vi "test_RPLiDAR_Main3.vi"() -> ()   [LabVIEW 2019]
uses:
  Ctrl/rplidar_cmd.ctl
panel:
  out "XY Graph 4":cluster{"X":dbl, "Y":dbl}[](graph)=[{"X"=0.2824515072806151, "Y"=0.6855971091208806}, {"X"=0.2973493100074656, "Y"=0.6926199898487512}, {"X"=0.3182824081797592, "Y"=0.6879391751043789}, {"X"=0.32968595340345086, "Y"=0.6878188239852538}, {"X"=0.37688086730076775, "Y"=0.6851896174509806}, {"X"=0.423959702735745, "Y"=0.6772438042951879}, {"X"=0.10556803270784879, "Y"=0.0575799702170344}, {"X"=0.12764458907753945, "Y"=0.07189651507010685}, {"X"=0.162706267337329, "Y"=0.09217196194696962}, {"X"=0.5750904329426066, "Y"=0.3543603306493057}, {"X"=1.029570390073907, "Y"=0.5877032090120513}, {"X"=1.0369879212881827, "Y"=0.5729647577315851}, {"X"=1.0389160564866784, "Y"=0.5542198819730025}, {"X"=1.030226109276704, "Y"=0.530956837948797}, {"X"=1.0296780247760362, "Y"=0.5126775085697838}, {"X"=1.022823338060012, "Y"=0.49026062621811095}, {"X"=1.025782655226549, "Y"=0.47458930322582177}, {"X"=1.0232750025025923, "Y"=0.45592579632361235}, {"X"=1.026310539216213, "Y"=0.4396122462963535}, {"X"=1.0220381799563654, "Y"=0.4207321252429865}, {"X"=1.0194214725289468, "Y"=0.40316736456081603}, {"X"=1.0201040780016217, "Y"=0.386164773826486}, {"X"=0.9777644288999799, "Y"=0.3543680594775664}, {"X"=0.981222843840791, "Y"=0.33935938652848674}, {"X"=0.9788143096363876, "Y"=0.32306053573756427}]
  out "x != 0?":bool
  in  "Boolean":bool
  in  "Tab Control":enum32{"UI", "ref"}(tab)
  out "buffer":u32(graph)
  in  "Reset":bool
  in  "port":refnum<visa-resource-name>="COM6"
  in  "baud rate":u32=115200
  in  "stop":bool
  out "dt_check":u32=20
  out "rs232 data":string
  in  "dt":u32=20
  out "response check":bool=TRUE
  out "n_enq":i32=10469
  out "n q buf":i32
  out "element":string
  in  "Reset data":bool=TRUE
  out "real packet":bool
  in  "scan":bool
  in  "health":bool
  in  "stop":bool
  in  "spin":bool
  out "health check":bool
  in  "close":bool
  out "XY Graph 3":cluster{"X":dbl, "Y":dbl}[](graph)=[{"X"=0.2824515072806151, "Y"=0.6855971091208806}, {"X"=0.2973493100074656, "Y"=0.6926199898487512}, {"X"=0.3182824081797592, "Y"=0.6879391751043789}, {"X"=0.32968595340345086, "Y"=0.6878188239852538}, {"X"=0.37688086730076775, "Y"=0.6851896174509806}, {"X"=0.423959702735745, "Y"=0.6772438042951879}, {"X"=0.10556803270784879, "Y"=0.0575799702170344}, {"X"=0.12764458907753945, "Y"=0.07189651507010685}, {"X"=0.162706267337329, "Y"=0.09217196194696962}, {"X"=0.5750904329426066, "Y"=0.3543603306493057}, {"X"=1.029570390073907, "Y"=0.5877032090120513}, {"X"=1.0369879212881827, "Y"=0.5729647577315851}, {"X"=1.0389160564866784, "Y"=0.5542198819730025}, {"X"=1.030226109276704, "Y"=0.530956837948797}, {"X"=1.0296780247760362, "Y"=0.5126775085697838}, {"X"=1.022823338060012, "Y"=0.49026062621811095}, {"X"=1.025782655226549, "Y"=0.47458930322582177}, {"X"=1.0232750025025923, "Y"=0.45592579632361235}, {"X"=1.026310539216213, "Y"=0.4396122462963535}, {"X"=1.0220381799563654, "Y"=0.4207321252429865}, {"X"=1.0194214725289468, "Y"=0.40316736456081603}, {"X"=1.0201040780016217, "Y"=0.386164773826486}, {"X"=0.9777644288999799, "Y"=0.3543680594775664}, {"X"=0.981222843840791, "Y"=0.33935938652848674}, {"X"=0.9788143096363876, "Y"=0.32306053573756427}]
  out "update":bool
  out "read buffer":string
  out "unsigned byte array 2":u8[][](array[numeric]) format="%02x"
  # "RPLIDAR"
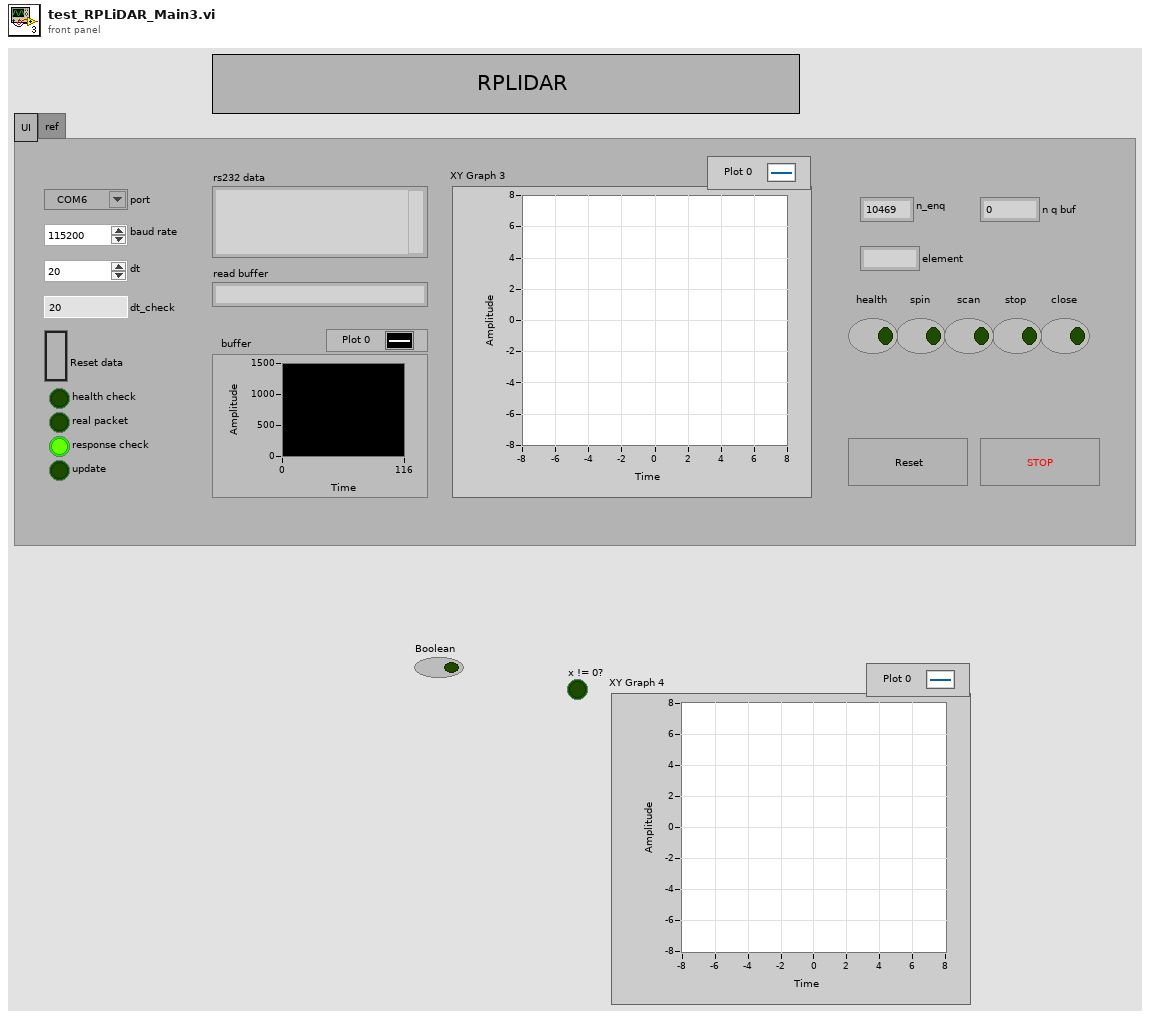
[diagram p1: front panel]
types:
  T1 = typedef "rplidar_cmd.ctl" = enum16{"init", "health", "spin", "scan", "read", "stop", "close"}
  T2 = cluster{"port":refnum<visa-resource-name>, "dt":u32, "update n":u8, "speed":u16, "rate ":u32}
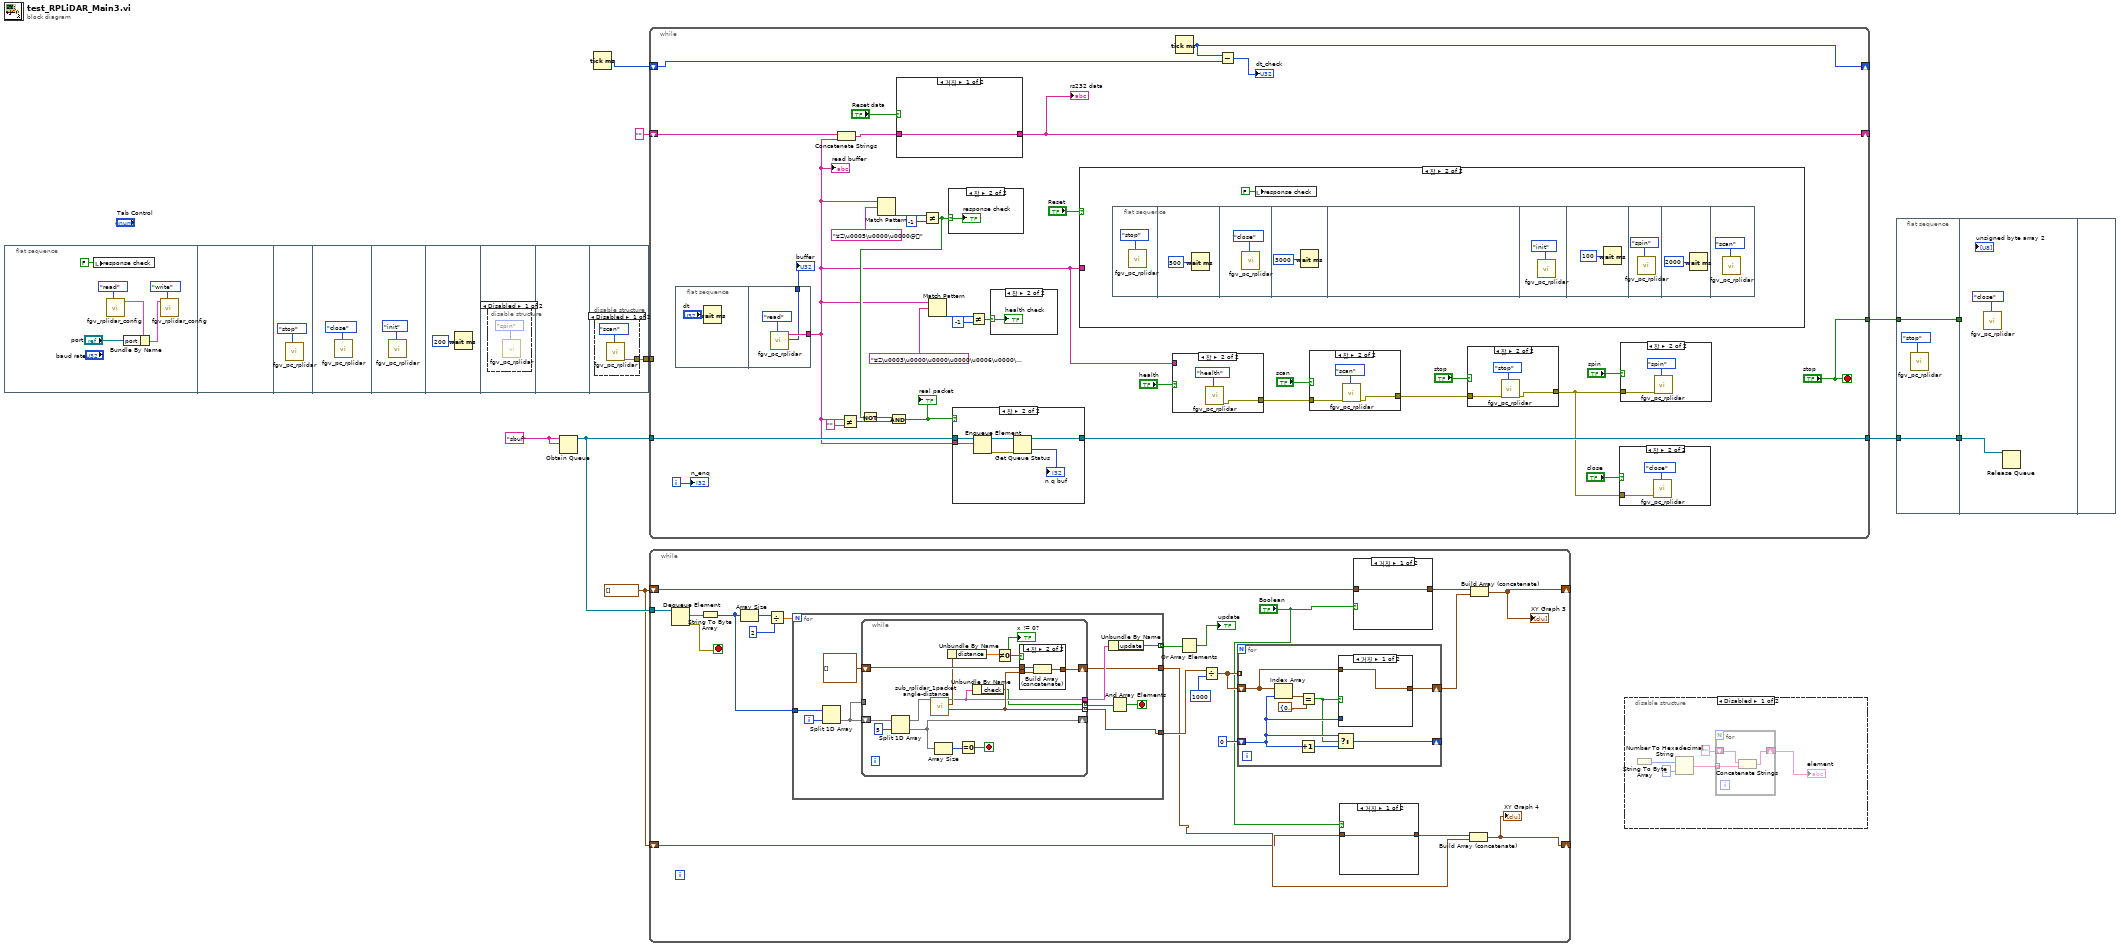
[diagram p0: block diagram]
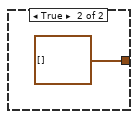
[diagram p3: hidden frame]
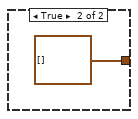
[diagram p4: hidden frame]
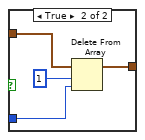
[diagram p5: hidden frame]
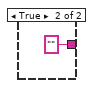
[diagram p15: hidden frame]
diagram:
  w1 = cluster{dbl, dbl}[] []
  w7 = "sbuf" ("name (unnamed)")
  n1 = flat-sequence {
    tunnel: [w22] -> w9
    frame #0 {
      n2 = local write "response check"(FALSE ("response check")) -> ()
      n3 = call "fgv_rplidar_config.vi"("cmd"=enum16{"read", "write"}."read") -> ("RPLidar cfg out"=w13:T2)  [unwired: 9 in, 1 out]
      n4 = Bundle By Name(cluster=w13, "port"="port") -> (w11:T2)
      n5 = call "fgv_rplidar_config.vi"("cmd"=enum16{"read", "write"}."write", "RPLidar cfg"=w11) -> ()  [unwired: 8 in, 2 out]
    }
    frame #1 {
    }
    frame #2 {
      n6 = call "fgv_pc_rplidar.vi"("cmd"=rplidar_cmd."stop") -> ()  [unwired: 8 in, 3 out]
    }
    frame #3 {
      n7 = call "fgv_pc_rplidar.vi"("cmd"=rplidar_cmd."close") -> ()  [unwired: 8 in, 3 out]
    }
    frame #4 {
      n8 = call "fgv_pc_rplidar.vi"("cmd"=rplidar_cmd."init") -> ()  [unwired: 8 in, 3 out]
    }
    frame #5 {
      n9 = Wait (ms)(milliseconds to wait=u32 200) -> ()  [unwired: 1 out]
    }
    frame #6 {
      n10 = disable-structure shown="Disabled" {
        frame Disabled {
          n11 = call "fgv_pc_rplidar.vi"("cmd"=rplidar_cmd."spin") -> ()  [unwired: 8 in, 3 out]
        }
        frame Enabled {
        }
      }
    }
    frame #7 {
    }
    frame #8 {
      n12 = disable-structure shown="Disabled" {
        disable-tunnel: [w23 _] -> w22
        frame Disabled {
          n13 = call "fgv_pc_rplidar.vi"("cmd"=rplidar_cmd."scan") -> ("error out"=w23:errorcluster)  [unwired: 8 in, 2 out]
        }
        frame Enabled {
        }
      }
    }
  }
  n14 = Obtain Queue(name (unnamed)=w7, element data type=w7) -> (queue out=w2:refnum<queue>)  [unwired: 3 in, 2 out]
  n15 = Tick Count (ms)() -> (millisecond timer value=w8:u32)
  n16 = while {
    tunnel: ["stop"] -> w10
    tunnel: w9 -> [_]
    shift-right: [w55] -> _
    shift-left: w8 -> [w54]
    shift-right: [w42] -> _
    shift-left: "" -> [w53]
    tunnel: w2 -> [w47]
    tunnel: [w46] -> w6
    i -> [w45]
    stop <- "stop" stop-if-true
    n17 = flat-sequence {
      tunnel: [w95] -> w28
      tunnel: [w93] -> w56
      frame #0 {
        n18 = Wait (ms)(milliseconds to wait="dt") -> ()  [unwired: 1 out]
      }
      frame #1 {
        n19 = call "fgv_pc_rplidar.vi"("cmd"=rplidar_cmd."read") -> ("serial buf"=w93:u32, "read buffer"=w95:string)  [unwired: 8 in, 1 out]
      }
    }
    n20 = Concatenate Strings(w53, w28) -> (w52:string)
    n21 = Not Equal?(x=w28, y="") -> (x != y?=w41:bool)
    n22 = Match Pattern(string=w28, regular expression="¥Z\u0005\u0000\u0000@") -> (offset past match=w50:i32)  [unwired: 1 in, 3 out]
    n23 = case shown="거짓" "Reset data" {
      tunnel: w52 -> [w72 _]
      tunnel: [w72 ""] -> w42
      frame False {
      }
      frame True {
      }
    }
    "rs232 data" <- w42
    n24 = Not Equal?(x=w50, y=-1) -> (x != y?=w40:bool)
    n25 = Not(x=w40) -> (.not. x?=w38:bool)
    n26 = And(x=w38, y=w41) -> (x .and. y?=w39:bool)
    "real packet" <- w39
    n27 = Match Pattern(string=w28, regular expression="¥Z\u0003\u0000\u0000\u0000\u0006\u0000\u0000\u0000") -> (offset past match=w30:i32)  [unwired: 1 in, 3 out]
    n28 = case shown="참" w40 {
      selector: w40 -> [_ w91]
      frame False {
      }
      frame True {
        "response check" <- w91
      }
    }
    n29 = case shown="참" w39 {
      tunnel: w47 -> [w74 w80]
      tunnel: [w74 w76] -> w46
      tunnel: w28 -> [_ w77]
      frame False {
      }
      frame True {
        n30 = Enqueue Element(queue=w80, element=w77) -> (queue out=w79:refnum<queue>, error out=w75:errorcluster)  [unwired: 2 in, 1 out]
        n31 = Get Queue Status(queue=w79, error in (no error)=w75) -> (queue out=w76:refnum<queue>, # elements in queue=→"n q buf":i32)  [unwired: 1 in, 6 out]
      }
    }
    n32 = Not Equal?(x=w30, y=-1) -> (x != y?=w32:bool)
    n33 = case shown="참" w32 {
      selector: w32 -> [_ w59]
      frame False {
      }
      frame True {
        "health check" <- w59
      }
    }
    n34 = case shown="참" "Reset" {
      tunnel: w28 -> [_ _]
      frame False {
      }
      frame True {
        n35 = flat-sequence {
          frame #0 {
            n36 = call "fgv_pc_rplidar.vi"("cmd"=rplidar_cmd."stop") -> ()  [unwired: 8 in, 3 out]
          }
          frame #1 {
            n37 = Wait (ms)(milliseconds to wait=u32 500) -> ()  [unwired: 1 out]
          }
          frame #2 {
            n38 = call "fgv_pc_rplidar.vi"("cmd"=rplidar_cmd."close") -> ()  [unwired: 8 in, 3 out]
          }
          frame #3 {
            n39 = Wait (ms)(milliseconds to wait=u32 3000) -> ()  [unwired: 1 out]
          }
          frame #4 {
          }
          frame #5 {
            n40 = call "fgv_pc_rplidar.vi"("cmd"=rplidar_cmd."init") -> ()  [unwired: 8 in, 3 out]
          }
          frame #6 {
            n41 = Wait (ms)(milliseconds to wait=u32 100) -> ()  [unwired: 1 out]
          }
          frame #7 {
            n42 = call "fgv_pc_rplidar.vi"("cmd"=rplidar_cmd."spin") -> ()  [unwired: 8 in, 3 out]
          }
          frame #8 {
            n43 = Wait (ms)(milliseconds to wait=u32 2000) -> ()  [unwired: 1 out]
          }
          frame #9 {
            n44 = call "fgv_pc_rplidar.vi"("cmd"=rplidar_cmd."scan") -> ()  [unwired: 8 in, 3 out]
          }
        }
        n45 = local write "response check"(FALSE ("response check")) -> ()
      }
    }
    n46 = case shown="참" "health" {
      tunnel: w28 -> [_ _]
      tunnel: [_ w70] -> w27
      frame False {
      }
      frame True {
        n47 = call "fgv_pc_rplidar.vi"("cmd"=rplidar_cmd."health") -> ("error out"=w70:errorcluster)  [unwired: 8 in, 2 out]
      }
    }
    n48 = Tick Count (ms)() -> (millisecond timer value=w55:u32)
    n49 = Subtract(x=w55, y=w54) -> (x-y=→"dt_check":u32)
    n50 = case shown="참" "scan" {
      tunnel: w27 -> [_ w68]
      tunnel: [_ w67] -> w26
      frame False {
      }
      frame True {
        n51 = call "fgv_pc_rplidar.vi"("cmd"=rplidar_cmd."scan", "error in"=w68) -> ("error out"=w67:errorcluster)  [unwired: 7 in, 2 out]
      }
    }
    n52 = case shown="참" "stop" {
      tunnel: w26 -> [_ w65]
      tunnel: [_ w64] -> w25
      frame False {
      }
      frame True {
        n53 = call "fgv_pc_rplidar.vi"("cmd"=rplidar_cmd."stop", "error in"=w65) -> ("error out"=w64:errorcluster)  [unwired: 7 in, 2 out]
      }
    }
    n54 = case shown="참" "close" {
      tunnel: w25 -> [_ w60]
      frame False {
      }
      frame True {
        n55 = call "fgv_pc_rplidar.vi"("cmd"=rplidar_cmd."close", "error in"=w60) -> ()  [unwired: 7 in, 3 out]
      }
    }
    n56 = case shown="참" "spin" {
      tunnel: w25 -> [_ w62]
      frame False {
      }
      frame True {
        n57 = call "fgv_pc_rplidar.vi"("cmd"=rplidar_cmd."spin", "error in"=w62) -> ()  [unwired: 7 in, 3 out]
      }
    }
    "buffer" <- w56
    "n_enq" <- w45
    "read buffer" <- w28
  }
  n58 = while {
    tunnel: w2 -> [w117]
    shift-right: [w102] -> _
    shift-left: w1 -> [w105]
    shift-right: [w97] -> _
    shift-left: w1 -> [w98]
    stop <- w116 stop-if-true
    n59 = Dequeue Element(queue=w117) -> (element=w115:string, error out=w116:errorcluster)  [unwired: 2 in, 2 out]
    n60 = String To Byte Array(string=w115) -> (unsigned byte array=w114:u8[])
    n61 = Array Size(array=w114) -> (size(s)=w113:i32)
    n62 = Divide(x=w113, y=2) -> (x/y=w111:dbl)
    n63 = for {
      N: w111 -> [_]
      tunnel: w114 -> [w142]
      tunnel: [w137] -> w110
      tunnel: [w139] -> w101 mode=indexing
      tunnel: [w136] -> w99
      i -> [w143]
      stop <- w144 stop-if-true
      n64 = Split 1D Array(array=w142, index=w143) -> (second subarray=w141:u8[])  [unwired: 1 out]
      n65 = while {
        tunnel: w141 -> [_]
        shift-right: [w157] -> _
        shift-left: w141 -> [w158]
        tunnel: [w150] -> w137 mode=indexing
        shift-right: [w151] -> w136
        shift-left: cluster{"x":dbl, "y":dbl}[] [] -> [w152]
        tunnel: [w146] -> w140
        tunnel: [w145] -> w138 mode=indexing
        stop <- w155 stop-if-true
        n66 = Split 1D Array(array=w158, index=5) -> (first subarray=w154:u8[], second subarray=w157:u8[])
        n67 = call "sub_rplidar_1packet angle-distance.vi"("packet"=w154) -> ("xy"=w150:cluster{"x":dbl, "y":dbl}, "angle distance"=w147:cluster{"angle":dbl, "distance":dbl}, "udate check"=w146:cluster{"update":bool, "check":bool})  [unwired: 8 in]
        n68 = Array Size(array=w157) -> (size(s)=w156:i32)
        n69 = Unbundle By Name(w147) -> ("distance"=w148:dbl)
        n70 = Equal To 0?(x=w156) -> (x = 0?=w155:bool)
        n71 = Unbundle By Name(w146) -> ("check"=w145:bool)
        n72 = Not Equal To 0?(x=w148) -> (x != 0?=w149:bool)
        "x != 0?" <- w149
        n73 = case shown="참" w149 {
          tunnel: w152 -> [w159 w162]
          tunnel: [w159 w161] -> w151
          tunnel: w150 -> [_ w160]
          frame False {
          }
          frame True {
            n74 = Build Array (concatenate)(w162, w160) -> (w161:cluster{"x":dbl, "y":dbl}[])
          }
        }
      }
      n75 = Unbundle By Name(w140) -> ("update"=w139:bool)
      n76 = And Array Elements(Boolean array=w138) -> (logical AND=w144:bool)
    }
    n77 = Or Array Elements(Boolean array=w101) -> (logical OR=→"update":bool)
    n78 = Divide(x=w110, y=1000) -> (x/y=w107:cluster{"x":dbl, "y":dbl}[])
    n79 = for {
      tunnel: w107 -> [_] mode=indexing
      shift-right: [w126] -> w106
      shift-left: w107 -> [w122]
      shift-right: [w125] -> _
      shift-left: 0 -> [w124]
      n80 = Index Array(array=w122, index=w124) -> (element=w129:cluster{"x":dbl, "y":dbl})
      n81 = Increment(x=w124) -> (x+1=w127:i32)
      n82 = Equal?(x=w129, y=cluster{dbl, dbl} {0.0, -0.0}) -> (x = y?=w123:bool)
      n83 = Select(t=w124, s=w123, f=w127) -> (s? t:f=w125:i32)
      n84 = case shown="거짓" w123 {
        tunnel: w122 -> [w130 w134]
        tunnel: [w130 w133] -> w126
        tunnel: w124 -> [_ w131]
        frame False {
        }
        frame True {
          n85 = Delete From Array(array=w134, length=1, index=w131) -> (array with subset deleted=w133:cluster{"x":dbl, "y":dbl}[])  [unwired: 1 out]
        }
      }
    }
    n86 = case shown="거짓" "Boolean" {
      tunnel: w98 -> [w118 _]
      tunnel: [w118 cluster{dbl, dbl}[] []] -> w100
      frame False {
      }
      frame True {
      }
    }
    n87 = case shown="거짓" "Boolean" {
      tunnel: w105 -> [w120 _]
      tunnel: [w120 cluster{dbl, dbl}[] []] -> w104
      frame False {
      }
      frame True {
      }
    }
    n88 = Build Array (concatenate)(w100, w99) -> (w97:cluster{"x":dbl, "y":dbl}[])
    "XY Graph 4" <- w97
    n89 = Build Array (concatenate)(w104, w106) -> (w102:cluster{"x":dbl, "y":dbl}[])
    "XY Graph 3" <- w102
  }
  n90 = disable-structure shown="Disabled" {
    frame Disabled {
      n91 = String To Byte Array() -> (unsigned byte array=w166:u8[])  [unwired: 1 in]
      n92 = Number To Hexadecimal String(1:i16 2 ("폭(-)"), 2:w166) -> (0:w165:string[])
      n93 = for {
        tunnel: w165 -> [w170] mode=indexing
        shift-right: [w168] -> w167
        shift-left: "" -> [w169]
        n94 = Concatenate Strings(w169, w170) -> (w168:string)
      }
      "element" <- w167
    }
    frame Enabled {
    }
  }
  n95 = flat-sequence {
    tunnel: w6 -> [w172]
    tunnel: w10 -> [w173]
    tunnel: [w173] -> w5
    tunnel: [w172] -> w4
    tunnel: w5 -> [_]
    tunnel: w4 -> [w174]
    frame #0 {
      n96 = call "fgv_pc_rplidar.vi"("cmd"=rplidar_cmd."stop") -> ()  [unwired: 8 in, 3 out]
    }
    frame #1 {
      n97 = call "fgv_pc_rplidar.vi"("cmd"=rplidar_cmd."close") -> ()  [unwired: 8 in, 3 out]
      n98 = Release Queue(queue=w174) -> ()  [unwired: 2 in, 3 out]
    }
    frame #2 {
    }
  }
